vi "PH_Cam_BaseClass.get Perferomance.vi"(0 "i ref in":refnum<vi>, 5 "error in (no error)":errorcluster) -> (14 "i ref out":refnum<vi>, 19 "error out":errorcluster)   [LabVIEW 2014, in "PH_Cam_BaseClass.lvlib"]
doc: "This VI measures the performance (frames per second, stores the time of the last token frame to the attributes and puts the result to the related GUI element. Since this procedure may take some time, it should be off by default."
uses:
  PH_Cam_BaseClass.lvlib
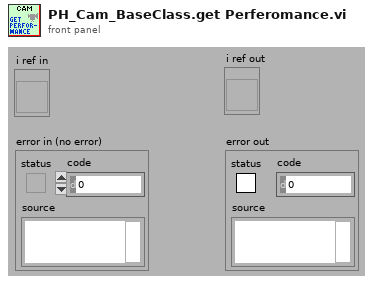
[diagram p1: front panel]
types:
  T1 = typedef "PH_Cam_BaseClass.lvlib/PH_Cam_BaseClass.i attribute.ctl" = cluster{"Gui Refs":T2, "Cam":cluster{"Source Notifier":refnum<notifier>, "Error":errorcluster, "Camera ID":string}, "Images":cluster{"Cam":T3, "Operation":T3, "PSDB":T3}, "Window Image":cluster{"Indicate Image":bool, "Window No.":i32, "Scale Facor":dbl, "Center Cross":bool, "Subtract Backgr":bool, "CoG":bool, "Color Palette":cluster{"Red":u8, "Green":u8, "Blue":u8}[], "Image On":bool}, "Default Prdc Int":i32, "Performance":cluster{"on":bool, "Timestamp Last Frame":i32}, "Histogram":cluster{"on":bool, "Mapping":bool}, "Save Image":cluster{"Save":bool, "File refnum":refnum<file>}, "Setting Service ID":i32, "Screen":cluster{"x-resolution":i16, "y-resolution":i16}, "On":bool, "Constructor finished":bool, "configured":bool}
  T2 = typedef "PH_Cam_BaseClass.lvlib/PH_Cam_BaseClass.GUI Refs.ctl" = cluster{"Frame Rate":refnum<vi>, "Get Frame Rate":refnum<vi>, "Show Image":refnum<vi>, "Get Histogram":refnum<vi>, "Mapping":refnum<vi>, "Histogram":refnum<vi>, "Center Cross":refnum<vi>, "Center of Gravity":refnum<vi>, "Scale Factor [%]":refnum<vi>, "Save Image":refnum<vi>, "Palette":refnum<vi>, "Subtract Background":refnum<vi>, "Cam Error":refnum<vi>, "On":refnum<vi>, "Cam List":refnum<vi>}
  T3 = typedef "IMAQ Image.ctl" = refnum<image>
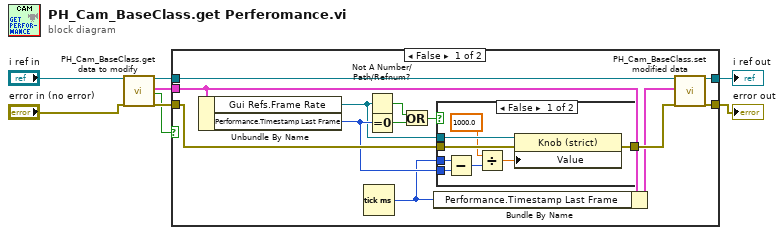
[diagram p0: block diagram]
diagram:
  n1 = call "PH_Cam_BaseClass.get data to modify.vi"("i ref in"="i ref in", "error in (no error)"="error in (no error)") -> ("i ref out"=w5:refnum<vi>, "i attribute"=w8:T1, "timed out"=w1:bool, "error out"=w7:errorcluster)  [unwired: 14 in]
  n2 = case shown="False" w1 {
    tunnel: w8 -> [w21 _]
    tunnel: w7 -> [w20 w31]
    tunnel: w5 -> [w19 w32]
    tunnel: [w11 w31] -> w3
    tunnel: [w10 w32] -> w2
    frame False {
      n3 = Unbundle By Name(w21) -> ("Gui Refs.Frame Rate"=w17:refnum<vi>, "Performance.Timestamp Last Frame"=w18:i32)
      n4 = Tick Count (ms)() -> (millisecond timer value=w9:u32)
      n5 = Not A Number/Path/Refnum?(number/path/refnum=w17) -> (NaN/Path/Refnum?=w16:bool)
      n6 = Equal To 0?(x=w18) -> (x = 0?=w15:bool)
      n7 = Or(x=w16, y=w15) -> (x .or. y?=w14:bool)
      n8 = Bundle By Name(cluster=w21, "Performance.Timestamp Last Frame"=w9) -> (w12:T1)
      n9 = case shown="False" w14 {
        tunnel: w20 -> [w29 w30]
        tunnel: [w28 w30] -> w13
        tunnel: w17 -> [w27 _]
        tunnel: w18 -> [w23 _]
        tunnel: w9 -> [w22 _]
        frame False {
          n10 = Subtract(x=w22, y=w23) -> (x-y=w25:u32)
          n11 = Divide(x=1000.0, y=w25) -> (x/y=w24:dbl)
          n12 = property class="Knob (strict)"(reference=w27, error in=w29, "Value"=w24) -> (error out=w28:errorcluster)  [unwired: 1 out]
        }
        frame True {
        }
      }
      n13 = call "PH_Cam_BaseClass.set modified data.vi"("i ref in"=w19, "i attribute"=w12, "error in (no error)"=w13) -> ("i ref out"=w10:refnum<vi>, "error out"=w11:errorcluster)  [unwired: 15 in]
    }
    frame True {
    }
  }
  "error out" <- w3
  "i ref out" <- w2
